vi "RSZVB Set Converter Data Set Type.vi"(8 "error in (no error)":errorcluster {"code" format="%.0x"}, 9 "Data Set Type (Factory Data Set)":i32(ring) items=["Factory Data Set", "User-Defined Data Set"], 10 "Port (1)":i32=1, 11 "VISA resource name":refnum<visa-resource-name>) -> (0 "error out":errorcluster {"code" format="%.0x"}, 3 "VISA resource name out":refnum<visa-resource-name>)   [LabVIEW 2011]
doc: "This VI specifies whether factory data or a user-defined data set shall be used.\n\nNote(s): \n\n(1) Use VI rszvb_SetSenseTypeOfPortTransferModel to set the Data Set mode.\n\nRemote-control command(s):\nSOURce<Ch>:POWer<Pt>:CONVerter:TRANsfer:DSET FACTory | USER"
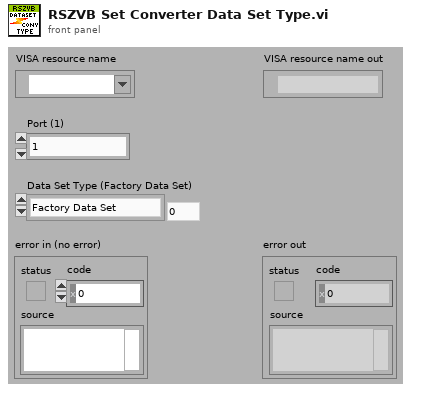
[diagram p1: front panel]
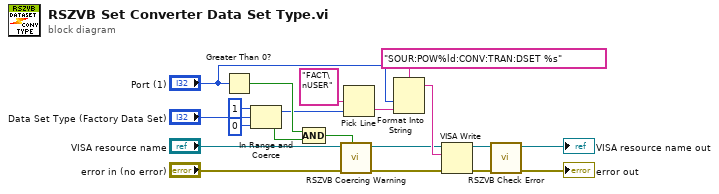
[diagram p0: block diagram]
diagram:
  n1 = Greater Than 0?(x="Port (1)") -> (x > 0?=w16:bool)
  n2 = In Range and Coerce(upper limit=1, x="Data Set Type (Factory Data Set)", lower limit=0) -> (coerced(x)=w9:i32, In Range?=w15:bool)
  n3 = Compound Arithmetic op=AND(w16, w15) -> (w17:bool)
  n4 = call "RSZVB Coercing Warning.vi"("In Range?"=w17, "error in (no error)"="error in (no error)", "VISA session"="VISA resource name") -> ("error out"=w11:errorcluster, "dup VISA session"=w10:refnum<visa-resource-name>)  [unwired: 7 in]
  n5 = Pick Line(multi-line string="FACT\nUSER", line index=w9) -> (output string=w14:string)  [unwired: 1 in]
  n6 = Format Into String(format string="SOUR:POW%ld:CONV:TRAN:DSET %s", "Port (1)", w14) -> (resulting string=w18:string)  [unwired: 2 in, 1 out]
  n7 = VISA Write(VISA resource name=w10, write buffer=w18, error in (no error)=w11) -> (VISA resource name out=w13:refnum<visa-resource-name>, error out=w12:errorcluster)  [unwired: 1 out]
  n8 = call "RSZVB Check Error.vi"("error in (no error)"=w12, "VISA session"=w13) -> ("error out"=→"error out":errorcluster, "dup VISA session"=→"VISA resource name out":refnum<visa-resource-name>)  [unwired: 8 in]
